vi "PH_Beckhoff_PP_Control.START PSDB THREADS.vi"(0 "VI in":refnum<vi>, 5 "error in (no error)":errorcluster) -> (14 "VI out":refnum<vi>, 19 "error out":errorcluster)   [LabVIEW 2014, in "PH_Beckhoff_PP_Control.lvlib"]
uses:
  PH_Beckhoff_PP_Control.lvlib
  CS_Core/CSSystem/CSSystemLib/CSSystemLib.lvlib
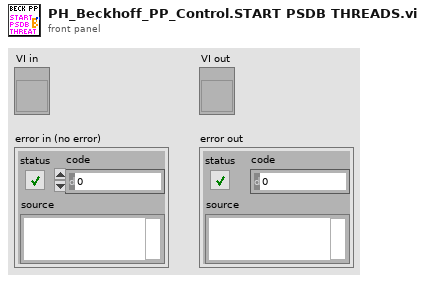
[diagram p1: front panel]
types:
  T1 = typedef "PH_Beckhoff_PP_Control.lvlib/PH_Beckhoff_PP_Control.i attribute.ctl" = cluster{"PP Conductivity Control":cluster{"PSDB":cluster{"Status Service ID":i32, "Instance ID":i32, "Data Status":T2, "Ref Status":refnum<vi>, "Error Code":i32}, "Status":cluster{"GUI Ref":refnum<vi>, "Status Service ID":i32, "Status":T3}, "DIs":cluster{"Device on":cluster{"GUI Ref":refnum<vi>, "# in Data":i32}, "Conductivity ok":cluster{"GUI Ref":refnum<vi>, "# in Data":i32}, "Temperature ok":cluster{"GUI Ref":refnum<vi>, "# in Data":i32}, "Alarm":cluster{"GUI Ref":refnum<vi>, "# in Data":i32}}, "PSDB Thread":cluster{"Ref":refnum<vi>, "Q-Ref":refnum<queue>}}, "PP Mercury Control":cluster{"PSDB":cluster{"Status Service ID":i32, "Instance ID":i32, "Data Status":T2, "Ref Status":refnum<vi>, "Error Code":i32}, "Status":cluster{"GUI Ref":refnum<vi>, "Status Service ID":i32, "Status":T3}, "on since:":cluster{"GUI Ref":refnum<vi>, "Service ID":i32, "Time":string}, "DIs":cluster{"Device on":cluster{"GUI Ref":refnum<vi>, "# in Data":i32}, "Alarm":cluster{"GUI Ref":refnum<vi>, "# in Data":i32}}, "AIs":cluster{"Concentration":cluster{"GUI Ref":refnum<vi>, "# in Data":i32}}, "PSDB Thread":cluster{"Ref":refnum<vi>, "Q-Ref":refnum<queue>}}, "PSDB":cluster{"Shot #":i32, "Subsystem":T4}, "PSDB Credentials":T5}
  T2 = typedef "PH_PSDBWriter.lvlib/PH_PSDBWriter.Data Status.ctl" = i16
  T3 = typedef "PH_StatusHandler.lvlib/PH_StatusHandler.Status.ctl" = i16
  T4 = typedef "PH_PSDBWriter.lvlib/PH_PSDBWriter.PHELIX-Subsystems.ctl" = i32
  T5 = typedef "PH_Common.lvlib/PH_Connection.PSDB Credentials.ctl" = cluster{"PW":string, "ID":string, "DS":string}
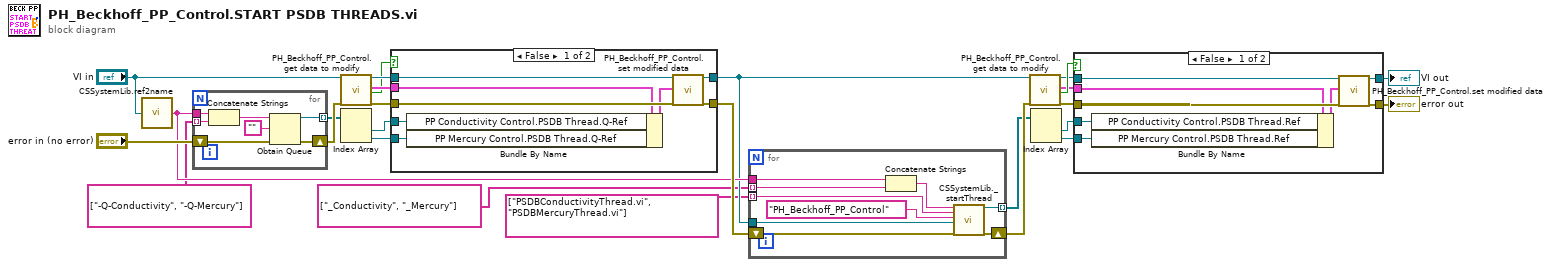
[diagram p0: block diagram]
diagram:
  n1 = call "CSSystemLib.ref2name.vi"("obj refnum"="VI in") -> ("name"=w11:string)
  n2 = for {
    tunnel: [w31] -> w24 mode=indexing
    tunnel: string[] ["-Q-Conductivity", "-Q-Mercury"] -> [w29] mode=indexing
    tunnel: w11 -> [w27]
    shift-right: [w33] -> w26
    shift-left: "error in (no error)" -> [w32]
    n3 = Concatenate Strings(w27, w29) -> (w30:string)
    n4 = Obtain Queue(name (unnamed)=w30, element data type="", error in (no error)=w32) -> (queue out=w31:refnum<queue>, error out=w33:errorcluster)  [unwired: 2 in, 1 out]
  }
  n5 = call "PH_Beckhoff_PP_Control.get data to modify.vi"("i ref in"="VI in", "error in (no error)"=w26) -> ("i ref out"=w22:refnum<vi>, "i attribute"=w20:T1, "timed out"=w19:bool, "error out"=w21:errorcluster)  [unwired: 14 in]
  n6 = Index Array(array=w24) -> (element #1=w9:refnum<queue>, element #2=w8:refnum<queue>)  [unwired: 2 in]
  n7 = case shown="False" w19 {
    tunnel: w22 -> [w41 w43]
    tunnel: [w40 w43] -> w6
    tunnel: w21 -> [w39 w42]
    tunnel: [w38 w42] -> w12
    tunnel: w20 -> [w37 _]
    tunnel: w9 -> [w35 _]
    tunnel: w8 -> [w34 _]
    frame False {
      n8 = Bundle By Name(cluster=w37, "PP Conductivity Control.PSDB Thread.Q-Ref"=w35, "PP Mercury Control.PSDB Thread.Q-Ref"=w34) -> (w36:T1)
      n9 = call "PH_Beckhoff_PP_Control.set modified data.vi"("i ref in"=w41, "i attribute"=w36, "error in (no error)"=w39) -> ("i ref out"=w40:refnum<vi>, "error out"=w38:errorcluster)  [unwired: 15 in]
    }
    frame True {
    }
  }
  n10 = for {
    tunnel: string[] ["PSDBConductivityThread.vi", "PSDBMercuryThread.vi"] -> [w52] mode=indexing
    tunnel: w11 -> [w49]
    tunnel: string[] ["_Conductivity", "_Mercury"] -> [w48] mode=indexing
    shift-right: [w46] -> w7
    shift-left: w12 -> [w51]
    tunnel: w6 -> [w45]
    tunnel: [w44] -> w5 mode=indexing
    n11 = Concatenate Strings(w49, w48) -> (w47:string)
    n12 = call "CSSystemLib._startThread.vi"("thread name"=w47, "template name"=w52, "Class"="PH_Beckhoff_PP_Control", "object ref"=w45, "error in (no error)"=w51) -> ("thread ref"=w44:refnum<vi>, "error out"=w46:errorcluster)  [unwired: 12 in, 1 out]
  }
  n13 = call "PH_Beckhoff_PP_Control.get data to modify.vi"("i ref in"=w6, "error in (no error)"=w7) -> ("i ref out"=w13:refnum<vi>, "i attribute"=w17:T1, "timed out"=w18:bool, "error out"=w15:errorcluster)  [unwired: 14 in]
  n14 = Index Array(array=w5) -> (element #1=w4:refnum<vi>, element #2=w3:refnum<vi>)  [unwired: 2 in]
  n15 = case shown="False" w18 {
    tunnel: w13 -> [w60 w62]
    tunnel: [w59 w62] -> w14
    tunnel: w15 -> [w58 w61]
    tunnel: [w57 w61] -> w16
    tunnel: w17 -> [w56 _]
    tunnel: w4 -> [w54 _]
    tunnel: w3 -> [w53 _]
    frame False {
      n16 = Bundle By Name(cluster=w56, "PP Conductivity Control.PSDB Thread.Ref"=w54, "PP Mercury Control.PSDB Thread.Ref"=w53) -> (w55:T1)
      n17 = call "PH_Beckhoff_PP_Control.set modified data.vi"("i ref in"=w60, "i attribute"=w55, "error in (no error)"=w58) -> ("i ref out"=w59:refnum<vi>, "error out"=w57:errorcluster)  [unwired: 15 in]
    }
    frame True {
    }
  }
  "error out" <- w16
  "VI out" <- w14
